vi "PNS Variabler Taktmerker II.vi"(8 "error in (no error)":errorcluster caption="Fehler (Eingang, kein Fehler)", 9 "Aus in sec.":dbl, 10 "Ein in sec.":dbl, 11 "Aktion":T1=enum."Lesen") -> (0 "error out":errorcluster caption="Fehler (Ausgang)", 2 "Takt":bool, 3 "Aktion":T1=enum."Lesen")   [LabVIEW 2015, in "PNS.lvlib"]
uses:
  PNS.lvlib
  Aktion PNS FGV variabler Taktmerker.ctl
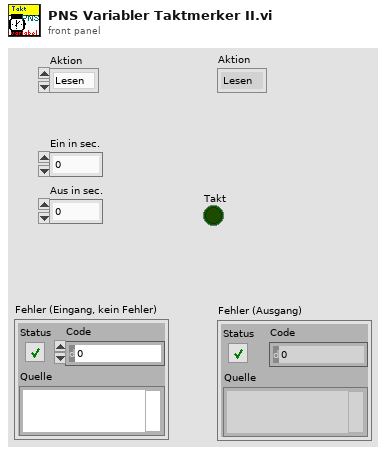
[diagram p1: front panel]
types:
  T1 = typedef "PNS.lvlib/Aktion PNS FGV variabler Taktmerker.ctl" = enum16{"Initialisieren", "Lesen", "aktiv", "inaktiv", "Werte schreiben"}
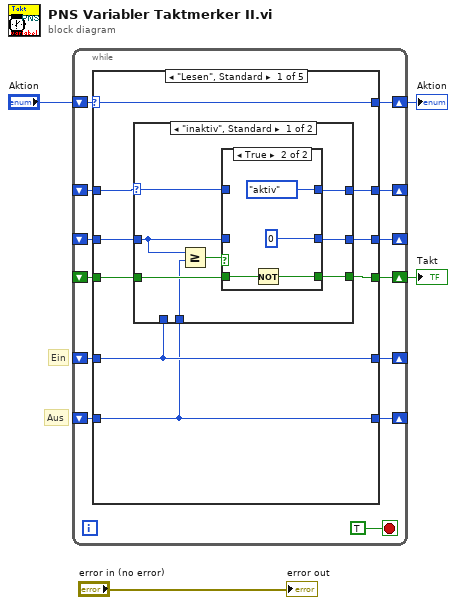
[diagram p0: block diagram]
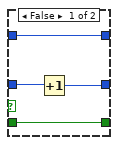
[diagram p2: hidden frame]
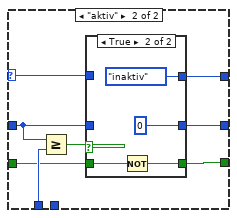
[diagram p3: hidden frame]
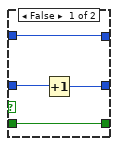
[diagram p4: hidden frame]
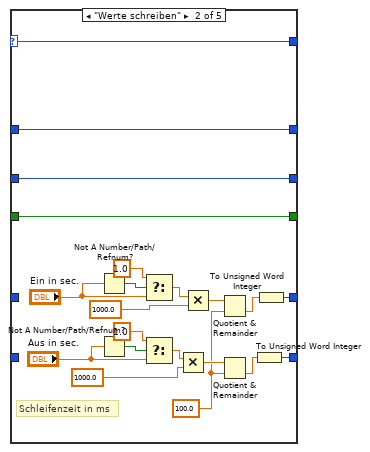
[diagram p5: hidden frame]
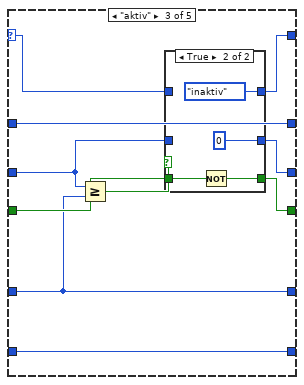
[diagram p6: hidden frame]
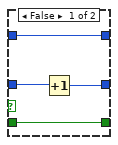
[diagram p7: hidden frame]
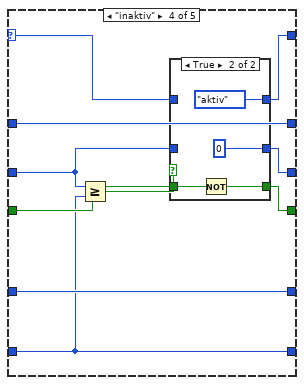
[diagram p8: hidden frame]
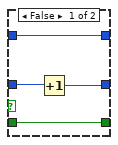
[diagram p9: hidden frame]
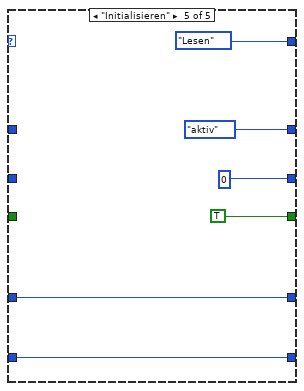
[diagram p10: hidden frame]
diagram:
  # "Aus"
  # "Ein"
  n1 = while {
    shift-right: [w15] -> _
    shift-left: _ -> [w14]
    shift-right: [w13] -> w2
    shift-left: _ -> [w12]
    shift-right: [w11] -> w3
    shift-left: "Aktion" -> [w16]
    shift-right: [w10] -> _
    shift-left: _ -> [w7]
    shift-right: [w9] -> _
    shift-left: _ -> [w8]
    shift-right: [w6] -> _
    shift-left: _ -> [w5]
    stop <- TRUE stop-if-true
    n2 = case shown="\"Lesen\", Standard" w16 {
      selector: w16 -> [w26 w79 w84 w102 _]
      tunnel: [w21 w78 w88 w106 u16 0 ("x+1")] -> w15
      tunnel: w14 -> [w22 w78 w87 w105 _]
      tunnel: [w23 w77 w86 w104 TRUE] -> w13
      tunnel: w12 -> [w24 w77 w85 w103 _]
      tunnel: [w26 w79 w83 w101 Aktion_PNS_FGV_variabler_Taktmerker."Lesen" ("Aktion")] -> w11
      tunnel: [w25 w69 w81 w100 w118] -> w10
      tunnel: [w18 w68 w82 w99 w117] -> w9
      tunnel: w8 -> [w18 _ w82 w99 w117]
      tunnel: w7 -> [w25 _ w81 w100 w118]
      tunnel: [w20 w59 w80 w98 Aktion_PNS_FGV_variabler_Taktmerker."aktiv" ("Aktion")] -> w6
      tunnel: w5 -> [w19 w59 w80 w98 _]
      frame "Lesen", Default {
        n3 = case shown="\"inaktiv\", Standard" w19 {
          selector: w19 -> [w27 w43]
          tunnel: w25 -> [_ w50]
          tunnel: w24 -> [w30 w49]
          tunnel: [w31 w48] -> w23
          tunnel: w22 -> [w29 w46]
          tunnel: [w32 w45] -> w21
          tunnel: [w33 w44] -> w20
          tunnel: w18 -> [w28 _]
          frame "inaktiv", Default {
            n4 = Greater Or Equal?(x=w29, y=w28) -> (x >= y?=w34:bool)
            n5 = case shown="True" w34 {
              tunnel: [w37 u16 0 ("x+1")] -> w32
              tunnel: w29 -> [w38 _]
              tunnel: [w36 w41] -> w31
              tunnel: w30 -> [w36 w40]
              tunnel: w27 -> [w35 _]
              tunnel: [w35 Aktion_PNS_FGV_variabler_Taktmerker."aktiv" ("Aktion")] -> w33
              frame False {
                n6 = Increment(x=w38) -> (x+1=w37:u16)
              }
              frame True {
                n7 = Not(x=w40) -> (.not. x?=w41:bool)
              }
            }
          }
          frame "aktiv" {
            n8 = Greater Or Equal?(x=w46, y=w50) -> (x >= y?=w47:bool)
            n9 = case shown="True" w47 {
              tunnel: [w53 u16 0 ("x+1")] -> w45
              tunnel: w46 -> [w54 _]
              tunnel: [w52 w57] -> w48
              tunnel: w49 -> [w52 w56]
              tunnel: [w51 Aktion_PNS_FGV_variabler_Taktmerker."inaktiv" ("Aktion")] -> w44
              tunnel: w43 -> [w51 _]
              frame False {
                n10 = Increment(x=w54) -> (x+1=w53:u16)
              }
              frame True {
                n11 = Not(x=w56) -> (.not. x?=w57:bool)
              }
            }
          }
        }
      }
      frame "Werte schreiben" {
        w71 = 100.0 ("y")
        # "Schleifenzeit in ms"
        n12 = Not A Number/Path/Refnum?(number/path/refnum="Ein in sec.") -> (NaN/Path/Refnum?=w67:bool)
        n13 = Not A Number/Path/Refnum?(number/path/refnum="Aus in sec.") -> (NaN/Path/Refnum?=w62:bool)
        n14 = Select(t=1.0, s=w67, f="Ein in sec.") -> (s? t:f=w64:dbl)
        n15 = Select(t=1.0, s=w62, f="Aus in sec.") -> (s? t:f=w61:dbl)
        n16 = Multiply(x=w61, y=1000.0) -> (x*y=w73:dbl)
        n17 = Multiply(x=w64, y=1000.0) -> (x*y=w74:dbl)
        n18 = Quotient & Remainder(x=w74, y=w71) -> (floor(x/y)=w72:dbl)  [unwired: 1 out]
        n19 = Quotient & Remainder(x=w73, y=w71) -> (floor(x/y)=w70:dbl)  [unwired: 1 out]
        n20 = To Unsigned Word Integer(number=w70) -> (unsigned 16bit integer=w68:u16)
        n21 = To Unsigned Word Integer(number=w72) -> (unsigned 16bit integer=w69:u16)
      }
      frame "aktiv" {
        n22 = Greater Or Equal?(x=w87, y=w81) -> (x >= y?=w89:bool)
        n23 = case shown="True" w89 {
          tunnel: [w92 u16 0 ("x+1")] -> w88
          tunnel: w87 -> [w93 _]
          tunnel: [w91 w96] -> w86
          tunnel: w85 -> [w91 w95]
          tunnel: w84 -> [w90 _]
          tunnel: [w90 Aktion_PNS_FGV_variabler_Taktmerker."inaktiv" ("Aktion")] -> w83
          frame False {
            n24 = Increment(x=w93) -> (x+1=w92:u16)
          }
          frame True {
            n25 = Not(x=w95) -> (.not. x?=w96:bool)
          }
        }
      }
      frame "inaktiv" {
        n26 = Greater Or Equal?(x=w105, y=w99) -> (x >= y?=w107:bool)
        n27 = case shown="True" w107 {
          tunnel: [w110 u16 0 ("x+1")] -> w106
          tunnel: w105 -> [w111 _]
          tunnel: [w109 w114] -> w104
          tunnel: w103 -> [w109 w113]
          tunnel: w102 -> [w108 _]
          tunnel: [w108 Aktion_PNS_FGV_variabler_Taktmerker."aktiv" ("Aktion")] -> w101
          frame False {
            n28 = Increment(x=w111) -> (x+1=w110:u16)
          }
          frame True {
            n29 = Not(x=w113) -> (.not. x?=w114:bool)
          }
        }
      }
      frame "Initialisieren" {
      }
    }
  }
  "Aktion" <- w3
  "Takt" <- w2
  "error out" <- "error in (no error)"
